vi "Pracownia4.vi"() -> ()   [LabVIEW 2019]
panel:
  out "Tablica":bool[](array[boolean])
  out "?":bool
  in  "?":enum16{"XOR", "OR", "AND"}(ring)
  in  "?":bool
  out "?":bool
  out "?":bool
  out "?":bool
  out "?":bool
  out "?":bool
  out "?":bool
  out "?":bool
  in  "?":bool
  in  "?":bool
  in  "?":bool
  in  "?":bool
  in  "?":bool
  in  "?":bool
  in  "?":bool
  in  "?":bool
  in  "?":bool
  in  "?":bool
  in  "?":bool
  in  "?":bool
  in  "?":bool
  in  "?":bool
  in  "?":bool
  in  "?":bool
  # "Bajt 1"
  # "Bajt 2"
  # "Wynik"
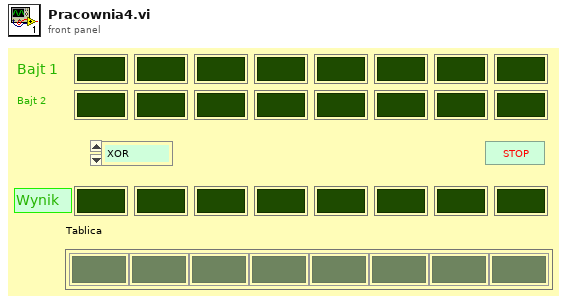
[diagram p1: front panel]
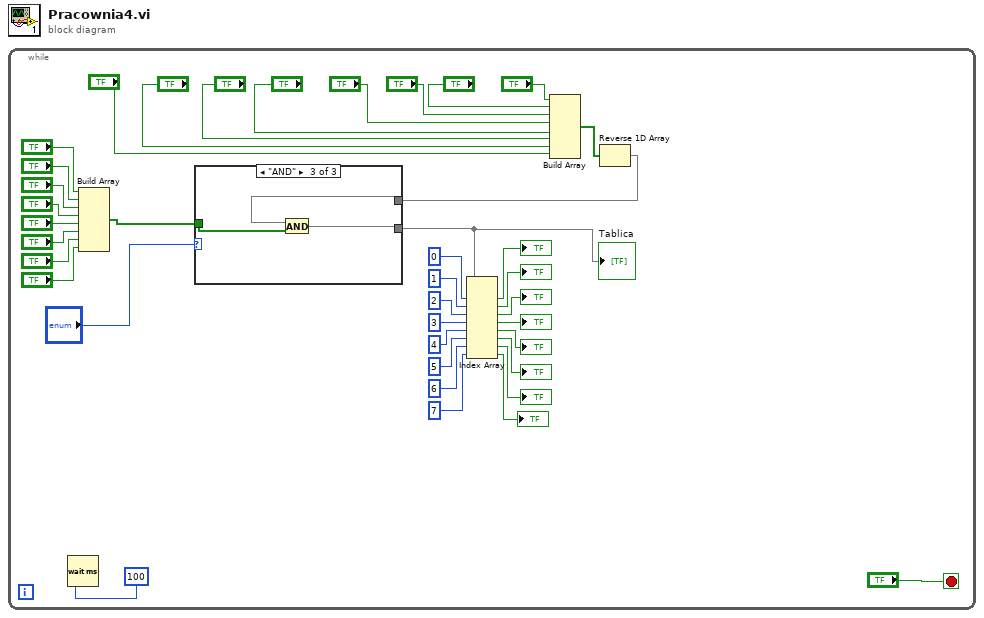
[diagram p0: block diagram]
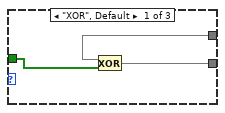
[diagram p2: hidden frame]
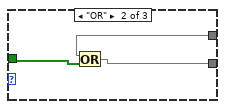
[diagram p3: hidden frame]
diagram:
  n1 = while {
    stop <- "?" stop-if-true
    n2 = Wait (ms)(milliseconds to wait=u32 100 ("millisecond timer value")) -> ()  [unwired: 1 out]
    n3 = Build Array("?", "?", "?", "?", "?", "?", "?", "?") -> (w21:bool[])
    n4 = Build Array("?", "?", "?", "?", "?", "?", "?", "?") -> (w3:bool[])
    n5 = Reverse 1D Array(array=w3) -> (reversed array=w2:bool[])
    n6 = case shown="\"AND\"" "?" {
      tunnel: w21 -> [w41 w45 w48]
      tunnel: w2 -> [w42 w43 w47]
      tunnel: [w40 w44 w46] -> w1
      frame "XOR", Default {
        n7 = Exclusive Or(1:w41, 2:w42) -> (0:w40:bool[])
      }
      frame "OR" {
        n8 = Or(x=w43, y=w45) -> (x .or. y?=w44:bool[])
      }
      frame "AND" {
        n9 = And(x=w47, y=w48) -> (x .and. y?=w46:bool[])
      }
    }
    "Tablica" <- w1
    n10 = Index Array(array=w1, index #1=0 ("index"), index #2=1 ("index"), index #3=2 ("index"), index #4=3 ("index"), index #5=4 ("index"), index #6=5 ("index"), index #7=6 ("index"), index #8=7 ("index")) -> (element #1=→"?":bool, element #2=→"?":bool, element #3=→"?":bool, element #4=→"?":bool, element #5=→"?":bool, element #6=→"?":bool, element #7=→"?":bool, element #8=→"?":bool)
  }
